vi "AutoDriveToBall.vi"(10 "Command Array":dbl[](array[numeric])) -> ()   [LabVIEW 2013]
uses:
  Drivetrain/Drivetrain Control.ctl
  Drivetrain/DT Mode.ctl
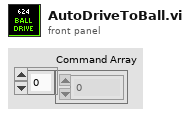
[diagram p1: front panel]
types:
  T1 = typedef "DT Mode.ctl" = enum16{"Manual", "Ball Steer", "Gyro Steer", "Goal Steer", "Fieldcentric", "Catch Steer", "Selfcatch", "Ball Drive", "Distance Drive"}
  T2 = typedef "Drivetrain Control.ctl" = cluster{"axis 1 (x)":dbl, "axis 2 (y)":dbl, "Mode":T1, "heading target":dbl, "steer axis":dbl, "omni?":bool, "Low Gear?":bool, "distance target":cluster{"x":dbl, "y":dbl}, "PID Params":cluster{"X Dist":cluster{"PID gains":cluster{"proportional gain (Kc)":dbl, "integral time (Ti, min)":dbl, "derivative time (Td, min)":dbl}, "output range":cluster{"output high":dbl, "output low":dbl}}, "Y Dist":cluster{"PID gains":cluster{"proportional gain (Kc)":dbl, "integral time (Ti, min)":dbl, "derivative time (Td, min)":dbl}, "output range":cluster{"output high":dbl, "output low":dbl}}}}
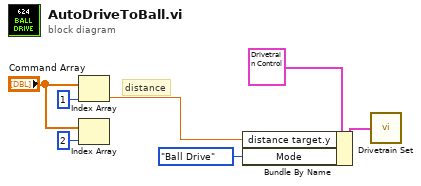
[diagram p0: block diagram]
diagram:
  # "distance"
  n1 = Index Array(array="Command Array", index=1) -> (element=w2:dbl)
  n2 = Index Array(array="Command Array", index=2) -> ()  [unwired: 1 out]
  n3 = Bundle By Name(cluster=T2 {"axis 1 (x)"=0.0, "axis 2 (y)"=0.0, "Mode"=enum."Manual", "heading target"=0.0, "steer axis"=0.0, "omni?"=FALSE, "Low Gear?"=FALSE, "distance target"={"x"=0.0, "y"=0.0}, "PID Params"={"X Dist"={"PID gains"={"proportional gain (Kc)"=1.0, "integral time (Ti, min)"=0.0, "derivative time (Td, min)"=0.0}, "output range"={"output high"=1.0, "output low"=-1.0}}, "Y Dist"={"PID gains"={"proportional gain (Kc)"=1.0, "integral time (Ti, min)"=0.0, "derivative time (Td, min)"=0.0}, "output range"={"output high"=1.0, "output low"=-1.0}}}} ("Drivetrain Control"), "distance target.y"=w2, "Mode"=DT_Mode."Ball Drive") -> (w4:T2)
  n4 = call "Drivetrain Set.vi"("Drivetrain Control"=w4) -> ()  [unwired: 1 in]
